vi "Demo RGB LED - Chaser With blinking onboard LED.vi"   [LabVIEW 2015]
doc: "This example demonstrates a theater light chaser on a 1-wire RGB LED strip using a WS2811 or WS2812 controller. The color of all LEDs can be preset on the front panel as well as the number of lights to cycle in the light chase. The time delay can also be adjusted to change the dramatic effect."
uses:
  <vilib>/Aledyne-TSXperts/Arduino Compatible Compiler for LabVIEW/Code Generator/Arduino APIs/Digital/PinDirection.ctl
  <vilib>/Aledyne-TSXperts/Arduino Compatible Compiler for LabVIEW/Code Generator/Arduino APIs/RGB LED Strip/RGB Strip Mode.ctl
  LED State.vi
  <vilib>/Aledyne-TSXperts/Arduino Compatible Compiler for LabVIEW/Arduino Compatible Compiler for LabVIEW.lvlib
panel:
  # "Overview: Demonstrates a theater light chaser on a 1-wire RGB LED strip using a WS2811 or WS2812 controller.  The color of all LEDs can be preset as well as the number of lights to cycle in the light chase.  The time delay can also be adjusted to change the dramatic effect.\n\nInstructions:\n1. Wire a 1-wire LED strip to a digital pin on the Arduino board.  Follow wiring instructions from the manufacturer.  A 100-500 ohm resistor is usually recommended between the Arduino digital output and the LED strip's data in pin.  Also, a 100 uF capacitor between the ground and power input may reduce noise on from the power supply.  It is also recommended to power the LED strip from a separate power input if available on the strip.  When daisy chaining LED strips, it is recommended to only daisy chain the Data line and to power each strip from a separate power input.\n2. Set the Digital Pin wired below.\n3. Set the Mode to the correct setting for your LED strip (the WS2812 uses 800kHz GRB).\n4. Set the Number of LEDs on your strip.  This can be set to any number equal to or smaller than the number of physical LEDs on the strip of you do not wish to power up all of them.\n5. Set Chase Every N Pixel to adjust how many pixels are moved on every cycle.\n6. Set the delay (ms) between LED rotations/shifts.\n7. Set the Red, Blue, and Green color of all LEDs on the strip.\n8.  If this example has been loaded from the Arduino Compatible Compiler for LabVIEW, simply select Compile and Download.  Otherwise, open Tools>Arduino Compatible Compiler for LabVIEW in LabVIEW, then select File>Load VI, and select this VI and then Compile and Download.\n9. Observe the LEDs on the strip as they appear to chase each other down the strip in a linear movement."
types:
  T1 = typedef "Arduino Compatible Compiler for LabVIEW.lvlib/RGB Strip Mode.ctl" = u16
  T2 = typedef "Arduino Compatible Compiler for LabVIEW.lvlib/PinDirection.ctl" = enum16{" INPUT", "OUTPUT", " INPUT_PULLUP"}
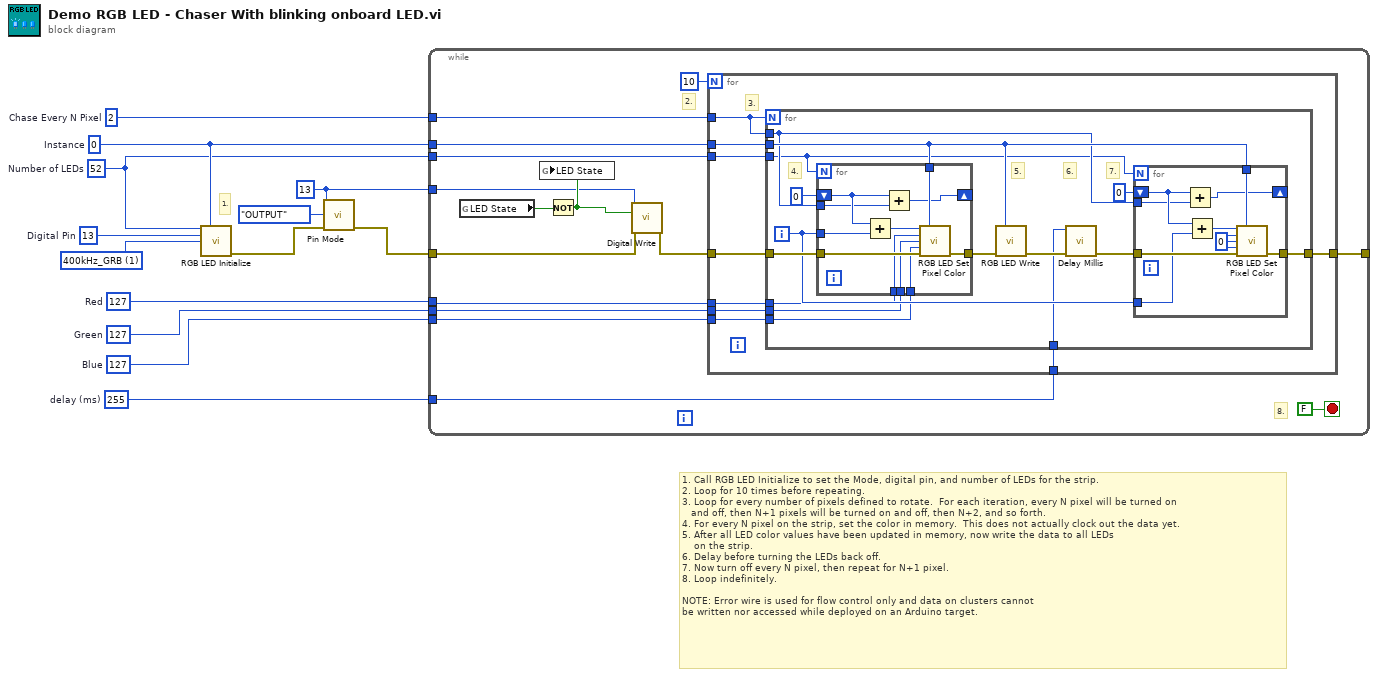
[diagram p0: block diagram]
diagram:
  w5 = u8 255  # delay (ms)
  w9 = u8 127  # Blue
  w10 = u8 127  # Green
  w11 = u8 127  # Red
  w13 = T1 1 items=["400kHz_RGB"=0, "400kHz_GRB"=1, "400kHz_BRG"=4, "800kHz_RGB"=2, "800kHz_GRB"=3, "400kHz_BRG"=6] ("Mode")
  w12 = u8 13  # Digital Pin
  w6 = u16 52  # Number of LEDs
  w7 = u8 2  # Chase Every N Pixel
  w1 = u8 13 ("pin")
  w8 = u8 0  # Instance
  # "1."
  # "1. Call RGB LED Initialize to set the Mode, digital pin, and number of LEDs for the strip.\n2. Loop for 10 times before repeating.\n3. Loop for every number of pixels defined to rotate.  For each iteration, every N pixel will be turned on\n   and off, then N+1 pixels will be turned on and off, then N+2, and so forth.\n4. For every N pixel on the strip, set the color in memory.  This does not actually clock out the data yet. \n5. After all LED color values have been updated in memory, now write the data to all LEDs\n    on the strip.\n6. Delay before turning the LEDs back off.\n7. Now turn off every N pixel, then repeat for N+1 pixel.\n8. Loop indefinitely.\n\nNOTE: Error wire is used for flow control only and data on clusters cannot\nbe written nor accessed while deployed on an Arduino target."
  n1 = call <vilib>:"RGB LED Initialize.vi"("Number of Pixels"=w6, "Instance"=w8, "Pin"=w12, "Mode"=w13) -> ("error out"=w4:errorcluster)  [unwired: 11 in]
  n2 = call <vilib>:"Pin Mode.vi"("pin"=w1, "direction"=PinDirection."OUTPUT", "error in (no error)"=w4) -> ("error out"=w3:errorcluster)  [unwired: 12 in]
  n3 = while {
    tunnel: w3 -> [w15]
    tunnel: w11 -> [w21]
    tunnel: w10 -> [w20]
    tunnel: w9 -> [w19]
    tunnel: w8 -> [w26]
    tunnel: w7 -> [w25]
    tunnel: w6 -> [w24]
    tunnel: [w23] -> _
    tunnel: w5 -> [w22]
    tunnel: w1 -> [w16]
    stop <- FALSE stop-if-true
    # "8."
    # "2."
    n4 = global read "LED State.vi" "LED State"() -> (w18:bool)
    n5 = Not(x=w18) -> (.not. x?=w17:bool)
    n6 = global write "LED State.vi" "LED State"(w17) -> ()
    n7 = call <vilib>:"Digital Write.vi"("pin"=w16, "state"=w17, "error in (no error)"=w15) -> ("error out"=w14:errorcluster)  [unwired: 12 in]
    n8 = for {
      N: u16 10 ("Number of Pixels") -> [_]
      tunnel: w26 -> [w37]
      tunnel: w14 -> [w36]
      tunnel: w25 -> [w35]
      tunnel: w24 -> [w34]
      tunnel: [w33] -> w23
      tunnel: w22 -> [w32]
      tunnel: w21 -> [w31]
      tunnel: w20 -> [w30]
      tunnel: w19 -> [w29]
      # "3."
      n9 = for {
        N: w35 -> [_]
        tunnel: w37 -> [w48]
        tunnel: w36 -> [w51]
        tunnel: w35 -> [w44]
        tunnel: w34 -> [w43]
        tunnel: [w42] -> w33
        tunnel: w32 -> [w41]
        tunnel: w31 -> [w40]
        tunnel: w30 -> [w39]
        tunnel: w29 -> [w38]
        i -> [w47]
        # "7."
        # "6."
        # "5."
        # "4."
        n10 = for {
          N: w43 -> [_]
          tunnel: w48 -> [w72]
          tunnel: w47 -> [w71]
          tunnel: [w70] -> w52
          tunnel: w51 -> [w69]
          shift-right: [w68] -> _
          shift-left: u8 0 ("Number of Pixels") -> [w66]
          tunnel: w44 -> [w65]
          tunnel: w40 -> [w64]
          tunnel: w39 -> [w63]
          tunnel: w38 -> [w62]
          n11 = Add(x=w66, y=w71) -> (x+y=w67:i32)
          n12 = Add(x=w66, y=w65) -> (x+y=w68:u8)
          n13 = call <vilib>:"RGB LED Set Pixel Color.vi"("Pixel"=w67, "Instance"=w72, "Red"=w64, "Green"=w63, "Blue"=w62, "error in (no error)"=w69) -> ("error out"=w70:errorcluster)  [unwired: 9 in]
        }
        n14 = call <vilib>:"RGB LED Write.vi"("Instance"=w48, "error in (no error)"=w52) -> ("error out"=w50:errorcluster)  [unwired: 13 in]
        n15 = call <vilib>:"Delay Millis.vi"("error in (no error)"=w50, "delay"=w41) -> ("error out"=w49:errorcluster)  [unwired: 9 in]
        n16 = for {
          N: w43 -> [_]
          tunnel: w48 -> [w61]
          tunnel: [w59] -> w42
          tunnel: w49 -> [w58]
          tunnel: w47 -> [w56]
          shift-right: [w55] -> _
          shift-left: u8 0 ("Number of Pixels") -> [w54]
          tunnel: w44 -> [w53]
          w57 = u8 0 ("Red")
          n17 = Add(x=w54, y=w53) -> (x+y=w55:u8)
          n18 = Add(x=w54, y=w56) -> (x+y=w60:i32)
          n19 = call <vilib>:"RGB LED Set Pixel Color.vi"("Pixel"=w60, "Instance"=w61, "Red"=w57, "Green"=w57, "Blue"=w57, "error in (no error)"=w58) -> ("error out"=w59:errorcluster)  [unwired: 9 in]
        }
      }
    }
  }
